vi "Simple_Example_IMAQ.vi"() -> ()   [LabVIEW 2019]
doc: "This example shows a simple recording of an image sequence and the image access afterwards.\nIt is a good starting point for writing own applications.\nBut it will not be fail save, i.e. doesnt react on errors, just handles them forward to the end\n\nUsage:\nSelect your required image count before you start the program.\nOnce started, the camera class will be initialized and images will be recorded automatically.\nWhen acquisition has finished you can address the images and set a certain roi \nTo finish the program click on quit application, this will force fan exit of the camera class"
uses:
  camera/Camera.lvclass
panel:
  out "rawImage":u16[][](array[numeric])
  out "Image":T1(plugin-control)
  in  "data_format":T2(ring)=enum."Mono16"
  in  "Image Index":u32 max=99
  out "Recorded Images":u32
  in  "Quit":bool
  in  "cropY1":u64=2 min=2 max=1040 step=1
  in  "cropX1":u64=2 min=2 max=1392 step=1
  in  "cropY0":u64=1 min=1 max=1039 step=1
  in  "cropX0":u64=1 min=1 max=1391 step=1
  out "Image Height":u16
  out "Image Width":u16
  in  "dwImgCount":u32=10 caption="Required Number of Images" max=4023
  out "Error":errorcluster {"code" format="%x"}
  # "This example shows a simple recording of an image sequence and the image access afterwards.\nIt is a good starting point for writing own applications.\nBut it will not be fail save, i.e. doesnt react on errors, just handles them forward to the end\n\nUsage:\nSelect your required image count before you start the program.\nOnce started, the camera class will be initialized and images will be recorded automatically.\nWhen acquisition has finished you can address the images and crop them to a smaller size \nTo finish the program click on quit application, this will force fan exit of the camera class"
  # "pco.labview"
  # "Camera Setup"
  # "Recording Control"
  # "Parameters for image readout"
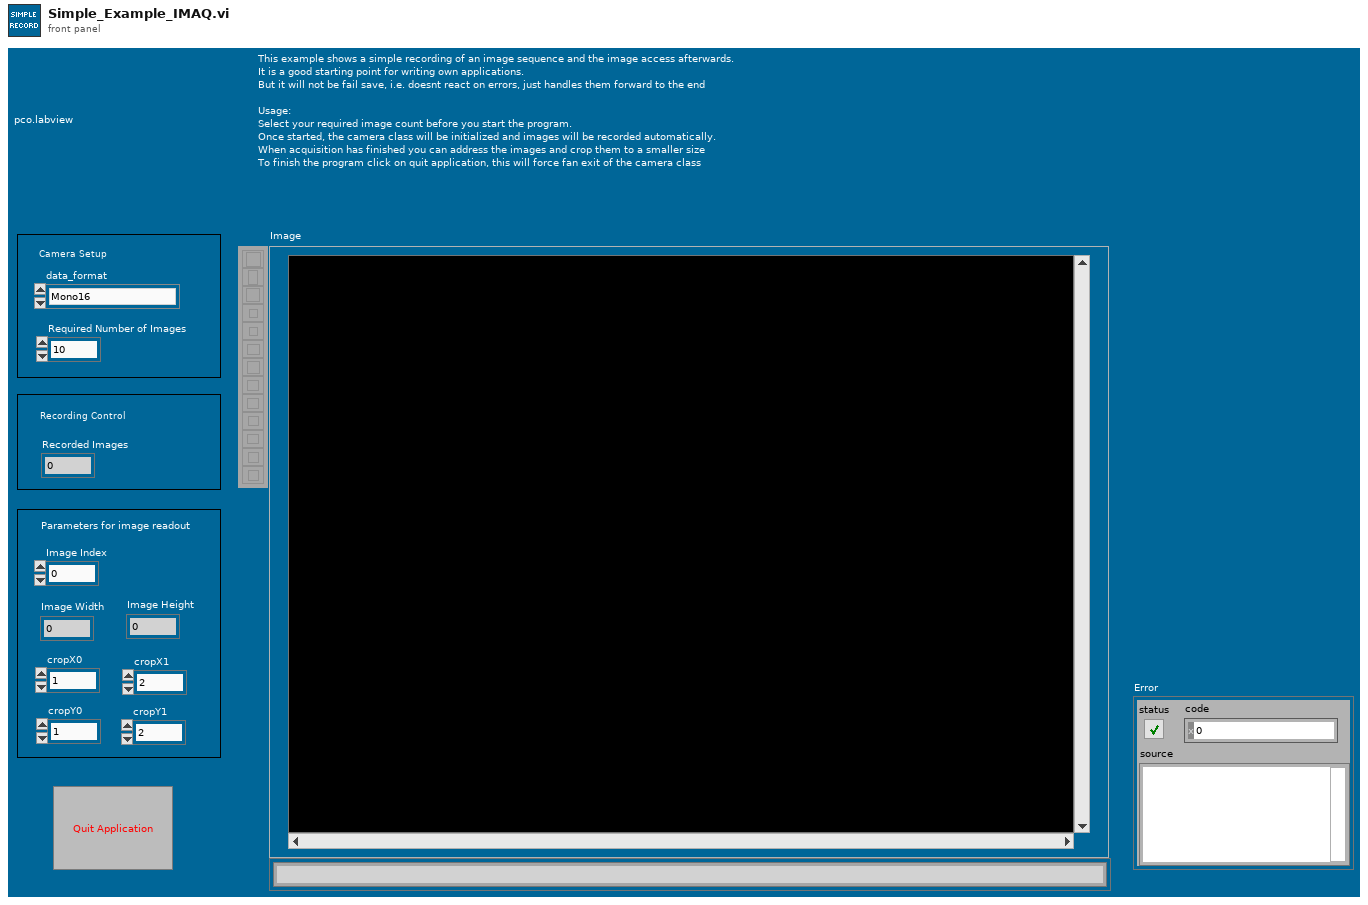
[diagram p1: front panel]
types:
  T1 = typedef "IMAQ Image.ctl" = refnum<image>
  T2 = enum16{"Undefined", "Mono8", "Mono16", "BGRA8", "RGBA8", "BGRA16", "RGBA16", "CompressedMono8"}
  T3 = enum8{"Enabled", "Disabled", "Disabled and Grayed Out"}
  T4 = enum16{"sequence", "sequence non blocking", "ring buffer", "fifo", "tif", "multitif", "pcoraw", "b16", "dicom", "multidicom", "camram_ring", "camram_segment"}
  T5 = cluster{"serial":u32, "type":u16, "sub_type":u16, "interface_type":u16, "bit_resolution":u16, "min_exposure_time_s":dbl, "max_exposure_time_s":dbl, "min_exposure_step_s":dbl, "min_delay_time_s":dbl, "max_delay_time_s":dbl, "min_delay_step_s":dbl, "min_width":u64, "min_height":u64, "max_width":u64, "max_height":u64, "roi_step_horz":u64, "roi_step_vert":u64, "roi_symmetric_horz":bool, "roi_symmetric_vert":bool, "has_timestamp_mode":bool, "has_timestamp_mode_ascii_only":bool, "pixelrate_vec":u32[], "conversion_factor_vec":sgl[], "has_trigger_mode_extexpctrl":bool, "has_acquire_mode":bool, "has_ext_acquire_mode":bool, "has_metadata_mode":bool, "has_ram":bool, "binning_horz_vec":u16[], "binning_vert_vec":u16[], "has_average_binning":bool, "pixel_format_vec":u32[]}
  T6 = typedef "Image Type" = u32
  T7 = typedef "Camera.lvclass/binning.ctl" = cluster{"vert":u16, "horz":u16, "mode":u16}
  T8 = cluster{"exposure_time_s":dbl, "delay_time_s":dbl, "roi":cluster{"x0":u64, "y0":u64, "x1":u64, "y1":u64}, "timestamp_mode":u16, "pixelrate":u32, "conversion_factor":sgl, "trigger_mode":u16, "acquire_mode":u16, "acquire_sequence_number":u32, "metadata_mode":u16, "noisefilter_mode":u16, "pixel_format":u32, "binning":T7, "auto_exposure":cluster{"region":u16, "min_exposure_s":dbl, "max_exposure_s":dbl}}
  T9 = cluster{"Plane 4 (alpha)":u16, "Plane 1 (Red)":u16, "Plane 2 (Green)":u16, "Plane 3 (Blue)":u16}[][]
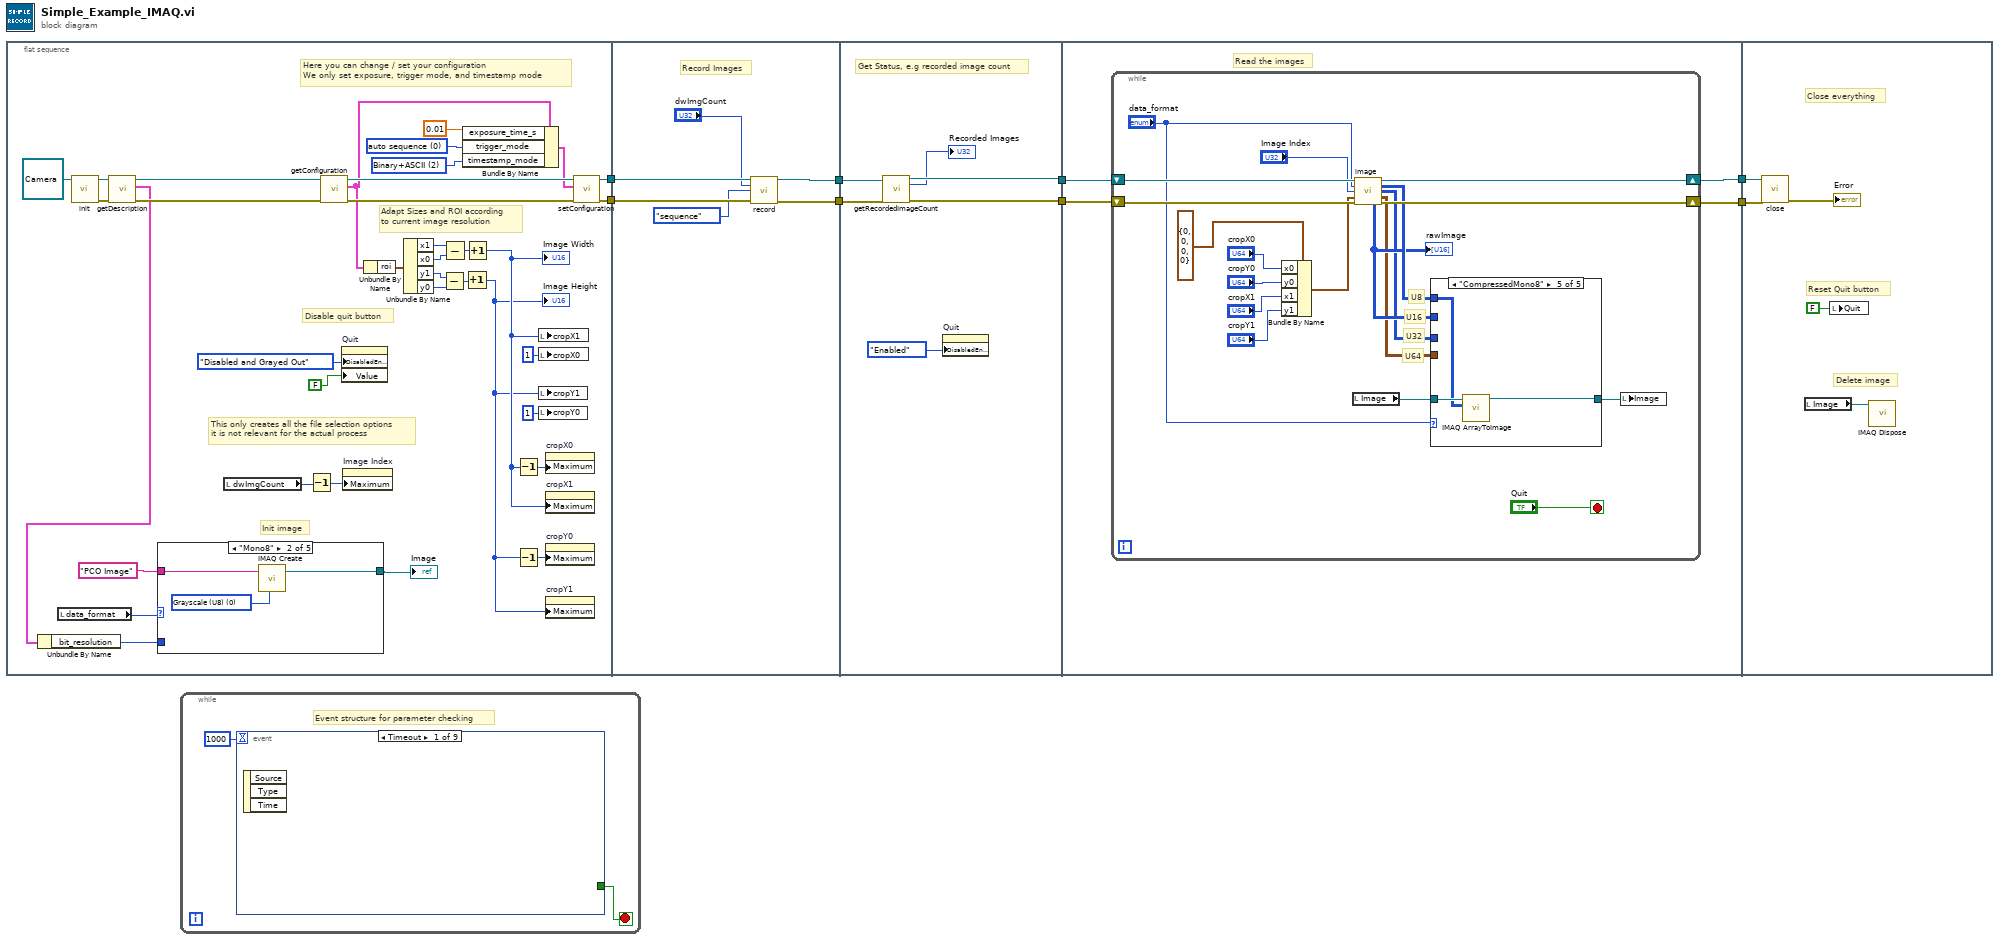
[diagram p0: block diagram]
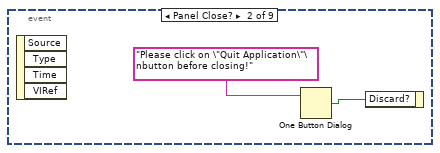
[diagram p2: hidden frame]
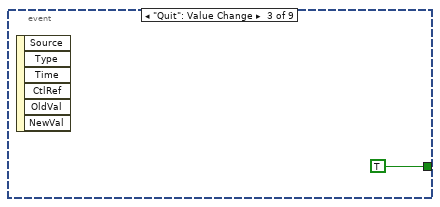
[diagram p3: hidden frame]
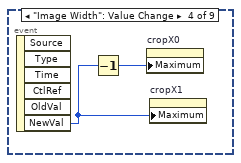
[diagram p4: hidden frame]
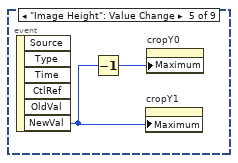
[diagram p5: hidden frame]
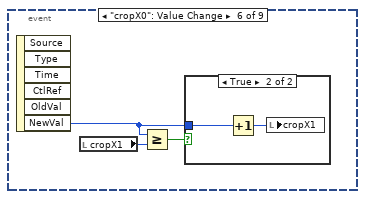
[diagram p6: hidden frame]
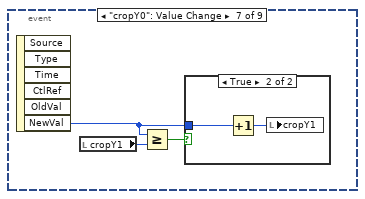
[diagram p8: hidden frame]
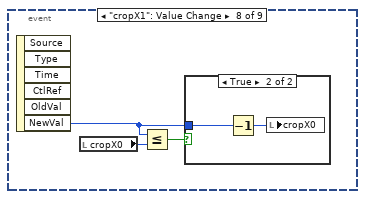
[diagram p10: hidden frame]
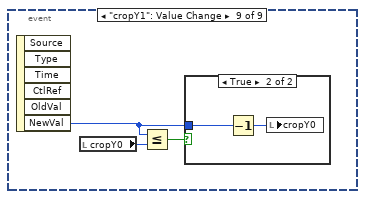
[diagram p12: hidden frame]
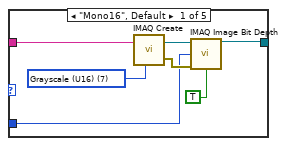
[diagram p14: hidden frame]
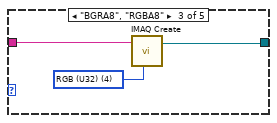
[diagram p15: hidden frame]
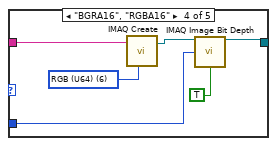
[diagram p16: hidden frame]
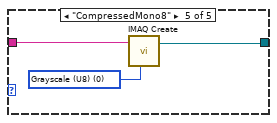
[diagram p17: hidden frame]
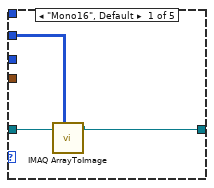
[diagram p18: hidden frame]
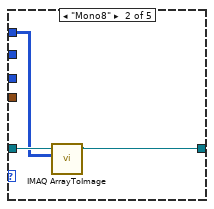
[diagram p19: hidden frame]
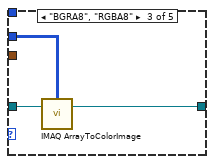
[diagram p20: hidden frame]
diagram:
  n1 = flat-sequence {
    tunnel: [w39] -> w8
    tunnel: [w38] -> w7
    tunnel: w8 -> [w72]
    tunnel: w7 -> [w71]
    tunnel: [w69] -> w6
    tunnel: [w68] -> w5
    tunnel: w6 -> [w78]
    tunnel: w5 -> [w77]
    tunnel: [w76] -> w4
    tunnel: [w75] -> w3
    tunnel: w4 -> [w81]
    tunnel: w3 -> [w82]
    tunnel: [w80] -> w2
    tunnel: [w79] -> w1
    tunnel: w2 -> [w119]
    tunnel: w1 -> [w118]
    frame #0 {
      w23 = u16 2 items=["OFF", "Binary", "Binary+ASCII", "ASCII"] ("TimestampMode")
      w43 = u16 0 items=["auto sequence"=0, "software trigger"=1, "external exposure start & software trigger"=2, "external exposure control"=3, "external synchronized"=4, "fast external exposure control"=5, "external CDS control"=6, "slow external exposure control"=7, "external synchronized HDSDI"=258] ("TriggerMode")
      # "Here you can change / set your configuration\nWe only set exposure, trigger mode, and timestamp mode"
      # "Init image"
      # "This only creates all the file selection options\nit is not relevant for the actual process"
      # "Adapt Sizes and ROI according\nto current image resolution"
      # "Disable quit button"
      n2 = local read "data_format"() -> (w18:T2)
      n3 = call-dynamic "init.vi"("Camera in"=refnum<class "Camera.lvclass"> refnum ("PCOCamera in")) -> ("Camera out"=w14:refnum<class "Camera.lvclass">, "error out"=w15:errorcluster)  [unwired: 8 in]
      n4 = call-dynamic "getDescription.vi"("error in (no error)"=w15, "Camera in"=w14) -> ("error out"=w12:errorcluster, "description"=w11:T5, "Camera out"=w13:refnum<class "Camera.lvclass">)  [unwired: 7 in]
      n5 = Unbundle By Name(w11) -> ("bit_resolution"=w10:u16)
      n6 = case shown="\"Mono8\"" w18 {
        tunnel: "PCO Image" ("Image Name") -> [w50 w54 w56 w62 w65]
        tunnel: [w46 w52 w55 w59 w64] -> w17
        tunnel: w10 -> [w45 _ _ w58 _]
        frame "Mono16", Default {
          w51 = T6 7 items=["Grayscale (U8)", "Grayscale (I16)", "Grayscale (SGL)", "Complex (CSG)", "RGB (U32)", "HSL (U32)", "RGB (U64)", "Grayscale (U16)"] ("Image Type")
          n7 = call "IMAQ Create"("Image Name"=w50, "Image Type"=w51) -> ("New Image"=w48:T1, "error out"=w47:errorcluster)  [unwired: 3 in]
          n8 = call "IMAQ Image Bit Depth"("Image"=w48, "Bit Depth (0)"=w45, "error in (no error)"=w47, "Get/Set Bit Depth? (Set)"=TRUE) -> ("Image Out"=w46:T1)  [unwired: 9 in, 2 out]
        }
        frame "Mono8" {
          w53 = T6 0 items=["Grayscale (U8)", "Grayscale (I16)", "Grayscale (SGL)", "Complex (CSG)", "RGB (U32)", "HSL (U32)", "RGB (U64)", "Grayscale (U16)"] ("Image Type")
          n9 = call "IMAQ Create"("Image Name"=w54, "Image Type"=w53) -> ("New Image"=w52:T1)  [unwired: 3 in, 1 out]
        }
        frame "BGRA8", "RGBA8" {
          w57 = T6 4 items=["Grayscale (U8)", "Grayscale (I16)", "Grayscale (SGL)", "Complex (CSG)", "RGB (U32)", "HSL (U32)", "RGB (U64)", "Grayscale (U16)"] ("Image Type")
          n10 = call "IMAQ Create"("Image Name"=w56, "Image Type"=w57) -> ("New Image"=w55:T1)  [unwired: 3 in, 1 out]
        }
        frame "BGRA16", "RGBA16" {
          w63 = T6 6 items=["Grayscale (U8)", "Grayscale (I16)", "Grayscale (SGL)", "Complex (CSG)", "RGB (U32)", "HSL (U32)", "RGB (U64)", "Grayscale (U16)"] ("Image Type")
          n11 = call "IMAQ Create"("Image Name"=w62, "Image Type"=w63) -> ("New Image"=w60:T1)  [unwired: 3 in, 1 out]
          n12 = call "IMAQ Image Bit Depth"("Image"=w60, "Bit Depth (0)"=w58, "Get/Set Bit Depth? (Set)"=TRUE) -> ("Image Out"=w59:T1)  [unwired: 10 in, 2 out]
        }
        frame "CompressedMono8" {
          w66 = T6 0 items=["Grayscale (U8)", "Grayscale (I16)", "Grayscale (SGL)", "Complex (CSG)", "RGB (U32)", "HSL (U32)", "RGB (U64)", "Grayscale (U16)"] ("Image Type")
          n13 = call "IMAQ Create"("Image Name"=w65, "Image Type"=w66) -> ("New Image"=w64:T1)  [unwired: 3 in, 1 out]
        }
      }
      "Image" <- w17
      n14 = local read "dwImgCount"() -> (w19:u32)
      n15 = Decrement(x=w19) -> (x-1=w20:u32)
      n16 = call-dynamic "getConfiguration.vi"("error in (no error)"=w12, "Camera in"=w13) -> ("error out"=w41:errorcluster, "configuration"=w33:T8, "Camera out"=w42:refnum<class "Camera.lvclass">)  [unwired: 7 in]
      n17 = property on="Quit" class="Bool (strict)"("DisabledEnum"=T3."Disabled and Grayed Out" ("Disabled"), "Value"=FALSE ("Stop")) -> ()  [unwired: 2 in, 2 out]
      n18 = property on="Image Index" class="DigNum (strict)"("Maximum"=w20) -> ()  [unwired: 2 in, 2 out]
      n19 = Unbundle By Name(w33) -> ("roi"=w32:cluster{"x0":u64, "y0":u64, "x1":u64, "y1":u64})
      n20 = Unbundle By Name(w32) -> ("x1"=w30:u64, "x0"=w31:u64, "y1"=w28:u64, "y0"=w29:u64)
      n21 = Subtract(x=w28, y=w29) -> (x-y=w26:u64)
      n22 = Subtract(x=w30, y=w31) -> (x-y=w27:u64)
      n23 = Bundle By Name(cluster=w33, "exposure_time_s"=0.01, "trigger_mode"=w43, "timestamp_mode"=w23) -> (w40:T8)
      n24 = Increment(x=w26) -> (x+1=w24:u64)
      "Image Height" <- w24
      n25 = Increment(x=w27) -> (x+1=w25:u64)
      "Image Width" <- w25
      n26 = Decrement(x=w25) -> (x-1=w35:u64)
      n27 = Decrement(x=w24) -> (x-1=w34:u64)
      n28 = local write "cropX1"(w25) -> ()
      n29 = local write "cropX0"(u16 1 ("roiY0")) -> ()
      n30 = local write "cropY1"(w24) -> ()
      n31 = local write "cropY0"(u16 1 ("roiY0")) -> ()
      n32 = property on="cropX0" class="DigNum (strict)"("Maximum"=w35) -> ()  [unwired: 2 in, 2 out]
      n33 = property on="cropX1" class="DigNum (strict)"("Maximum"=w25) -> ()  [unwired: 2 in, 2 out]
      n34 = property on="cropY0" class="DigNum (strict)"("Maximum"=w34) -> ()  [unwired: 2 in, 2 out]
      n35 = property on="cropY1" class="DigNum (strict)"("Maximum"=w24) -> ()  [unwired: 2 in, 2 out]
      n36 = call-dynamic "setConfiguration.vi"("error in (no error)"=w41, "configuration"=w40, "Camera in"=w42) -> ("error out"=w38:errorcluster, "Camera out"=w39:refnum<class "Camera.lvclass">)  [unwired: 7 in]
    }
    frame #1 {
      # "Record Images"
      n37 = call-dynamic "record.vi"("Camera in"=w72, "num_images"="dwImgCount", "record_mode"=T4."sequence", "error in (no error)"=w71) -> ("Camera out"=w69:refnum<class "Camera.lvclass">, "error out"=w68:errorcluster)  [unwired: 10 in]
    }
    frame #2 {
      # "Get Status, e.g recorded image count"
      n38 = call-dynamic "getRecordedImageCount.vi"("Camera in"=w78, "error in (no error)"=w77) -> ("Camera out"=w76:refnum<class "Camera.lvclass">, "recorded_image_count"=→"Recorded Images":u32, "error out"=w75:errorcluster)  [unwired: 11 in]
      n39 = property on="Quit" class="Bool (strict)"("DisabledEnum"=T3."Enabled" ("Disabled")) -> ()  [unwired: 2 in, 2 out]
    }
    frame #3 {
      # "Read the images"
      n40 = while {
        shift-right: [w99] -> w80
        shift-left: w81 -> [w101]
        shift-right: [w94] -> w79
        shift-left: w82 -> [w100]
        stop <- "Quit" stop-if-true
        # "U64"
        # "U32"
        # "U16"
        # "U8"
        n41 = Bundle By Name(cluster=cluster{"x0":u64, "y0":u64, "x1":u64, "y1":u64} {"x0"=0, "y0"=0, "x1"=0, "y1"=0} ("roi"), "x0"="cropX0", "y0"="cropY0", "x1"="cropX1", "y1"="cropY1") -> (w93:cluster{"x0":u64, "y0":u64, "x1":u64, "y1":u64})
        n42 = local read "Image"() -> (w86:T1)
        n43 = call-dynamic "image.vi"("Camera in"=w101, "data_format"="data_format", "image_index"="Image Index", "crop"=w93, "error in (no error)"=w100) -> ("Camera out"=w99:refnum<class "Camera.lvclass">, "image (U8)"=w90:u8[][], "image (U32)"=w88:u32[][], "image (U64)"=w87:T9, "raw_image (U16)"=w89:u16[][], "error out"=w94:errorcluster)  [unwired: 2 in, 3 out]
        "rawImage" <- w89
        n44 = case shown="\"CompressedMono8\"" "data_format" {
          tunnel: w86 -> [w104 w107 w110 w113 w116]
          tunnel: [w102 w105 w109 w111 w115] -> w85
          tunnel: w87 -> [_ _ _ w112 _]
          tunnel: w88 -> [_ _ w108 _ _]
          tunnel: w90 -> [_ w106 _ _ w114]
          tunnel: w89 -> [w103 _ _ _ _]
          frame "Mono16", Default {
            n45 = call "IMAQ ArrayToImage"("Image Pixels (U16)"=w103, "Image"=w104) -> ("Image Out"=w102:T1)  [unwired: 8 in, 1 out]
          }
          frame "Mono8" {
            n46 = call "IMAQ ArrayToImage"("Image Pixels (U8)"=w106, "Image"=w107) -> ("Image Out"=w105:T1)  [unwired: 8 in, 1 out]
          }
          frame "BGRA8", "RGBA8" {
            n47 = call "IMAQ ArrayToColorImage"("Image Pixels (U32)"=w108, "Image"=w110) -> ("Image Out"=w109:T1)  [unwired: 3 in, 1 out]
          }
          frame "BGRA16", "RGBA16" {
            n48 = call "IMAQ ArrayToColorImage"("Image"=w113, "Image Pixels (U64)"=w112) -> ("Image Out"=w111:T1)  [unwired: 3 in, 1 out]
          }
          frame "CompressedMono8" {
            n49 = call "IMAQ ArrayToImage"("Image Pixels (U8)"=w114, "Image"=w116) -> ("Image Out"=w115:T1)  [unwired: 8 in, 1 out]
          }
        }
        n50 = local write "Image"(w85) -> ()
      }
    }
    frame #4 {
      # "Delete image"
      # "Reset Quit button"
      # "Close everything"
      n51 = call-dynamic "close.vi"("error in (no error)"=w118, "Camera in"=w119) -> ("error out"=→"Error":errorcluster)  [unwired: 9 in]
      n52 = local read "Image"() -> (w117:T1)
      n53 = local write "Quit"(FALSE ("Stop")) -> ()
      n54 = call "IMAQ Dispose"("Image"=w117) -> ()  [unwired: 5 in, 1 out]
    }
  }
  n55 = while {
    stop <- w122 stop-if-true
    # "Event structure for parameter checking"
    n56 = event shown="[0] Timeout" {
      selector: _ -> [_ _ _ _ _ _ _ _ _]
      dyn-events: _ -> [_ _ _ _ _ _ _ _ _]
      timeout: 1000 -> [_ _ _ _ _ _ _ _ _]
      tunnel: [_ _ TRUE _ _ _ _ _ _] -> w122
      event Timeout {
        n57 = event-data() -> ()  [unwired: 1 in, 3 out]
      }
      event Panel Close? {
        n58 = event-data() -> ()  [unwired: 1 in, 4 out]
        n59 = One Button Dialog(message="Please click on \"Quit Application\"\nbutton before closing!") -> (true=w124:bool)  [unwired: 1 in]
        n60 = event-data("Discard?"=w124) -> ()  [unwired: 1 in, 1 out]
      }
      event "Quit": Value Change {
        n61 = event-data() -> ()  [unwired: 1 in, 6 out]
      }
      event "Image Width": Value Change {
        n62 = event-data() -> ("NewVal"=w127:u16)  [unwired: 1 in, 5 out]
        n63 = Decrement(x=w127) -> (x-1=w128:u16)
        n64 = property on="cropX0" class="DigNum (strict)"("Maximum"=w128) -> ()  [unwired: 2 in, 2 out]
        n65 = property on="cropX1" class="DigNum (strict)"("Maximum"=w127) -> ()  [unwired: 2 in, 2 out]
      }
      event "Image Height": Value Change {
        n66 = event-data() -> ("NewVal"=w129:u16)  [unwired: 1 in, 5 out]
        n67 = Decrement(x=w129) -> (x-1=w130:u16)
        n68 = property on="cropY1" class="DigNum (strict)"("Maximum"=w129) -> ()  [unwired: 2 in, 2 out]
        n69 = property on="cropY0" class="DigNum (strict)"("Maximum"=w130) -> ()  [unwired: 2 in, 2 out]
      }
      event "cropX0": Value Change {
        n70 = event-data() -> ("NewVal"=w131:u64)  [unwired: 1 in, 5 out]
        n71 = local read "cropX1"() -> (w133:u64)
        n72 = Greater Or Equal?(x=w131, y=w133) -> (x >= y?=w132:bool)
        n73 = case shown="True" w132 {
          tunnel: w131 -> [_ w135]
          frame False {
          }
          frame True {
            n74 = Increment(x=w135) -> (x+1=w134:u64)
            n75 = local write "cropX1"(w134) -> ()
          }
        }
      }
      event "cropY0": Value Change {
        n76 = event-data() -> ("NewVal"=w136:u64)  [unwired: 1 in, 5 out]
        n77 = local read "cropY1"() -> (w138:u64)
        n78 = Greater Or Equal?(x=w136, y=w138) -> (x >= y?=w137:bool)
        n79 = case shown="True" w137 {
          tunnel: w136 -> [_ w140]
          frame False {
          }
          frame True {
            n80 = Increment(x=w140) -> (x+1=w139:u64)
            n81 = local write "cropY1"(w139) -> ()
          }
        }
      }
      event "cropX1": Value Change {
        n82 = event-data() -> ("NewVal"=w141:u64)  [unwired: 1 in, 5 out]
        n83 = local read "cropX0"() -> (w143:u64)
        n84 = Less Or Equal?(x=w141, y=w143) -> (x <= y?=w142:bool)
        n85 = case shown="True" w142 {
          tunnel: w141 -> [_ w145]
          frame False {
          }
          frame True {
            n86 = Decrement(x=w145) -> (x-1=w144:u64)
            n87 = local write "cropX0"(w144) -> ()
          }
        }
      }
      event "cropY1": Value Change {
        n88 = event-data() -> ("NewVal"=w146:u64)  [unwired: 1 in, 5 out]
        n89 = local read "cropY0"() -> (w148:u64)
        n90 = Less Or Equal?(x=w146, y=w148) -> (x <= y?=w147:bool)
        n91 = case shown="True" w147 {
          tunnel: w146 -> [_ w150]
          frame False {
          }
          frame True {
            n92 = Decrement(x=w150) -> (x-1=w149:u64)
            n93 = local write "cropY0"(w149) -> ()
          }
        }
      }
    }
  }
